vi "TrianglePlaneIntersect.vi"(10 "CuttingZ":sgl, 11 "TriangleFace":T3) -> (2 "Intersects?":bool, 3 "Line2D":T1)   [LabVIEW 2014]
uses:
  TypeDefs/TriangleFace.ctl
  TypeDefs/Point3D.ctl
  TypeDefs/Line2D.ctl
  TypeDefs/Point2DwSlope.ctl
  TypeDefs/Line3D.ctl
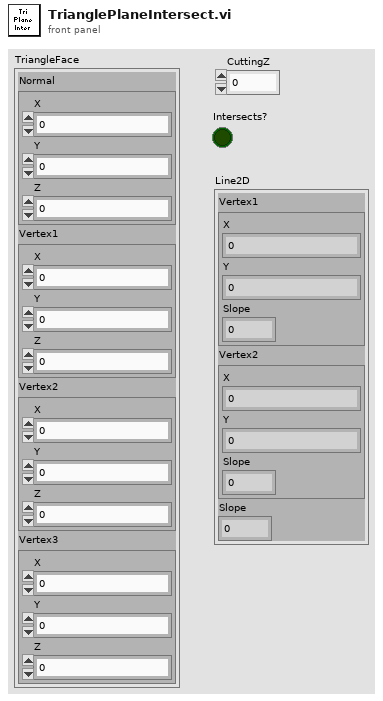
[diagram p1: front panel]
types:
  T1 = typedef "Line2D.ctl" = cluster{"Vertex1":T2, "Vertex2":T2, "Slope":dbl}
  T2 = typedef "Point2DwSlope.ctl" = cluster{"X":sgl, "Y":sgl, "Slope":dbl}
  T3 = typedef "TriangleFace.ctl" = cluster{"Normal":T4, "Vertex1":T4, "Vertex2":T4, "Vertex3":T4}
  T4 = typedef "Point3D.ctl" = cluster{"X":sgl, "Y":sgl, "Z":sgl}
  T5 = typedef "Line3D.ctl" = cluster{"Vertex1":T4, "Vertex2":T4}
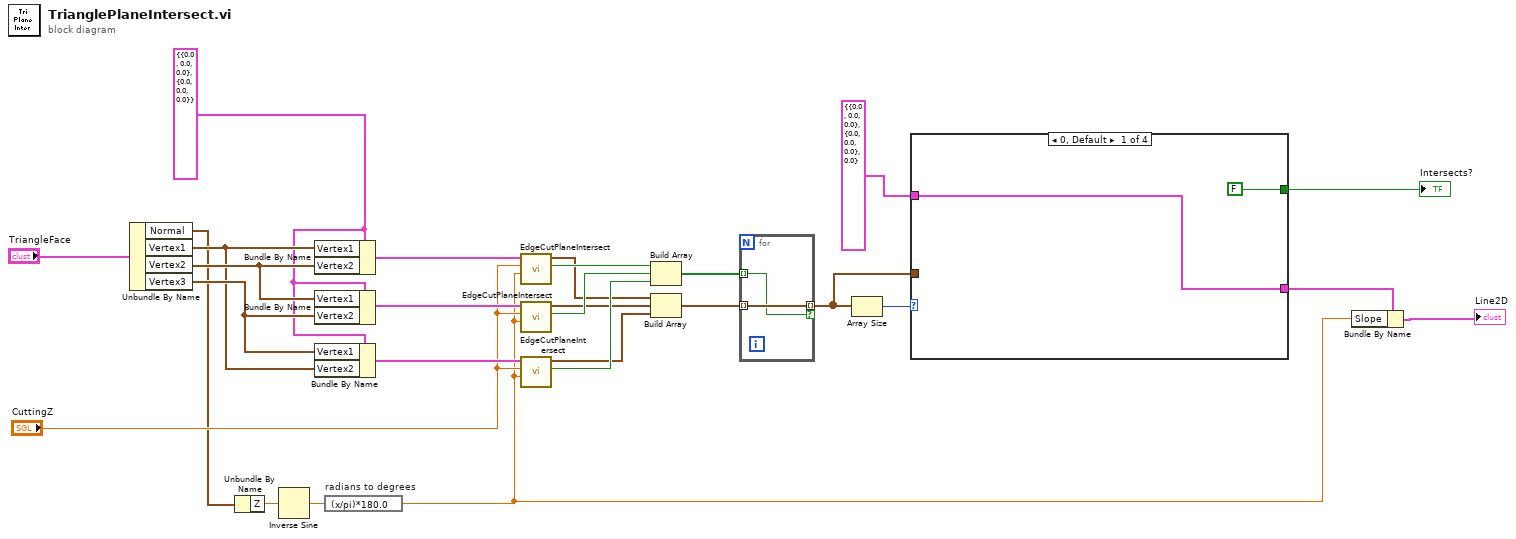
[diagram p0: block diagram]
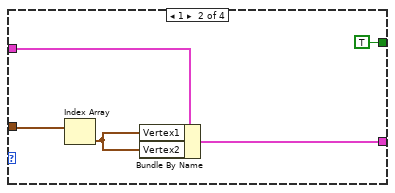
[diagram p2: hidden frame]
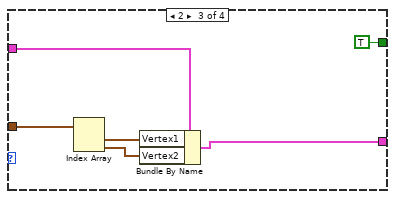
[diagram p3: hidden frame]
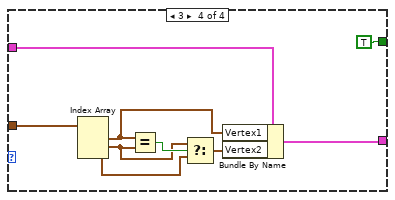
[diagram p4: hidden frame]
diagram:
  w23 = T5 {"Vertex1"={"X"=0.0, "Y"=0.0, "Z"=0.0}, "Vertex2"={"X"=0.0, "Y"=0.0, "Z"=0.0}} ("Line3D")
  n1 = Unbundle By Name("TriangleFace") -> ("Normal"=w6:T4, "Vertex1"=w24:T4, "Vertex2"=w26:T4, "Vertex3"=w25:T4)
  n2 = Unbundle By Name(w6) -> ("Z"=w5:sgl)
  n3 = Inverse Sine(1:w5) -> (0:w4:sgl)
  n4 = Bundle By Name(cluster=w23, "Vertex1"=w24, "Vertex2"=w26) -> (w22:T5)
  n5 = Bundle By Name(cluster=w23, "Vertex1"=w26, "Vertex2"=w25) -> (w21:T5)
  n6 = Bundle By Name(cluster=w23, "Vertex1"=w25, "Vertex2"=w24) -> (w20:T5)
  n7 = expression code="(x/pi)*180.0" "radians to degrees"(w4) -> (w1:sgl)
  n8 = call "EdgeCutPlaneIntersect.vi"("Slope"=w1, "CuttingZ"="CuttingZ", "Line3D"=w22) -> ("Intersect?"=w18:bool, "IntersectPoint"=w15:T2)  [unwired: 7 in]
  n9 = call "EdgeCutPlaneIntersect.vi"("Slope"=w1, "CuttingZ"="CuttingZ", "Line3D"=w21) -> ("Intersect?"=w17:bool, "IntersectPoint"=w14:T2)  [unwired: 7 in]
  n10 = call "EdgeCutPlaneIntersect.vi"("Slope"=w1, "CuttingZ"="CuttingZ", "Line3D"=w20) -> ("Intersect?"=w16:bool, "IntersectPoint"=w13:T2)  [unwired: 7 in]
  n11 = Build Array(w18, w17, w16) -> (w12:bool[])
  n12 = Build Array(w15, w14, w13) -> (w11:T2[])
  n13 = for {
    tunnel: w12 -> [w28] mode=indexing
    tunnel: w11 -> [w29] mode=indexing
    tunnel: [w29] -> w8 mode=indexing if=w28
  }
  n14 = Array Size(array=w8) -> (size(s)=w10:i32)
  n15 = case shown="0, Default" w10 {
    tunnel: [FALSE TRUE TRUE TRUE] -> w9
    tunnel: w8 -> [_ w36 w42 w50]
    tunnel: T1 {"Vertex1"={"X"=0.0, "Y"=0.0, "Slope"=0.0}, "Vertex2"={"X"=0.0, "Y"=0.0, "Slope"=0.0}, "Slope"=0.0} ("Line2D") -> [w30 w35 w41 w51]
    tunnel: [w30 w33 w38 w49] -> w3
    frame 0, Default {
    }
    frame 1 {
      n16 = Index Array(array=w36) -> (element=w34:T2)  [unwired: 1 in]
      n17 = Bundle By Name(cluster=w35, "Vertex1"=w34, "Vertex2"=w34) -> (w33:T1)
    }
    frame 2 {
      n18 = Index Array(array=w42) -> (element #1=w40:T2, element #2=w39:T2)  [unwired: 2 in]
      n19 = Bundle By Name(cluster=w41, "Vertex1"=w40, "Vertex2"=w39) -> (w38:T1)
    }
    frame 3 {
      n20 = Index Array(array=w50) -> (element #1=w46:T2, element #2=w45:T2, element #3=w44:T2)  [unwired: 3 in]
      n21 = Equal?(x=w46, y=w45) -> (x = y?=w47:bool)
      n22 = Select(t=w45, s=w47, f=w44) -> (s? t:f=w43:T2)
      n23 = Bundle By Name(cluster=w51, "Vertex1"=w46, "Vertex2"=w43) -> (w49:T1)
    }
  }
  "Intersects?" <- w9
  n24 = Bundle By Name(cluster=w3, "Slope"=w1) -> (→"Line2D":T1)
